vi "Velocity_Trajectory2.vi"() -> ()   [LabVIEW 2017]
uses:
  <vilib>/Analysis/1siggen.llb/Ramp Pattern by Samples.vi
  <vilib>/Analysis/NI_AALBase.lvlib
panel:
  in  "Max Velocity":dbl=2.0
  in  "Theta Final":dbl=100.0
  in  "Theta Initial":dbl=50.0
  out "Waveform Graph":dbl[](graph)=[0.0, 0.010101010101010102, 0.020202020202020204, 0.030303030303030304, 0.04040404040404041, 0.05050505050505051, 0.060606060606060615, 0.07070707070707072, 0.08080808080808081, 0.09090909090909091, 0.10101010101010101, 0.1111111111111111, 0.1212121212121212, 0.1313131313131313, 0.1414141414141414, 0.15151515151515152, 0.16161616161616163, 0.17171717171717174, 0.18181818181818185, 0.19191919191919196, 0.20202020202020207, 0.21212121212121218, 0.2222222222222223, 0.2323232323232324, 0.24242424242424251, 0.2525252525252526, 0.2626262626262627, 0.2727272727272728, 0.28282828282828293, 0.29292929292929304, 0.30303030303030315, 0.31313131313131326, 0.32323232323232337, 0.3333333333333335, 0.3434343434343436, 0.3535353535353537, 0.3636363636363638, 0.3737373737373739, 0.38383838383838403, 0.39393939393939414, 0.40404040404040426, 0.41414141414141437, 0.4242424242424245, 0.4343434343434346, 0.4444444444444447, 0.4545454545454548, 0.4646464646464649, 0.47474747474747503, 0.48484848484848514, 0.49494949494949525, 0.5050505050505053, 0.5151515151515154, 0.5252525252525254, 0.5353535353535355, 0.5454545454545455, 0.5555555555555556, 0.5656565656565656, 0.5757575757575757, 0.5858585858585857, 0.5959595959595958, 0.6060606060606059, 0.6161616161616159, 0.626262626262626, 0.636363636363636, 0.6464646464646461, 0.6565656565656561, 0.6666666666666662, 0.6767676767676762, 0.6868686868686863, 0.6969696969696964, 0.7070707070707064, 0.7171717171717165, 0.7272727272727265, 0.7373737373737366, 0.7474747474747466, 0.7575757575757567, 0.7676767676767667, 0.7777777777777768, 0.7878787878787868, 0.7979797979797969, 0.808080808080807, 0.818181818181817, 0.8282828282828271, 0.8383838383838371, 0.8484848484848472, 0.8585858585858572, 0.8686868686868673, 0.8787878787878773, 0.8888888888888874, 0.8989898989898975, 0.9090909090909075, 0.9191919191919176, 0.9292929292929276, 0.9393939393939377, 0.9494949494949477, 0.9595959595959578, 0.9696969696969678, 0.9797979797979779, 0.989898989898988, 0.999999999999998, 1.0, 1.0, 1.0, 1.0, 1.0, 1.0, 1.0, 1.0, 1.0, 1.0, 1.0, 1.0, 1.0, 1.0, 1.0, 1.0, 1.0, 1.0, 1.0, 1.0, 1.0, 1.0, 1.0, 1.0, 1.0, 1.0, 1.0, 1.0, 1.0, 1.0, 1.0, 1.0, 1.0, 1.0, 1.0, 1.0, 1.0, 1.0, 1.0, 1.0, 1.0, 1.0, 1.0, 1.0, 1.0, 1.0, 1.0, 1.0, 1.0, 1.0, 1.0, 1.0, 1.0, 1.0, 1.0, 1.0, 1.0, 1.0, 1.0, 1.0, 1.0, 1.0, 1.0, 1.0, 1.0, 1.0, 1.0, 1.0, 1.0, 1.0, 1.0, 1.0, 1.0, 1.0, 1.0, 1.0, 1.0, 1.0, 1.0, 1.0, 1.0, 1.0, 1.0, 1.0, 1.0, 1.0, 1.0, 1.0, 1.0, 1.0, 1.0, 1.0, 1.0, 1.0, 1.0, 1.0, 1.0, 1.0, 1.0, 1.0, 1.0, 0.98989898989899, 0.9797979797979799, 0.9696969696969698, 0.9595959595959598, 0.9494949494949497, 0.9393939393939397, 0.9292929292929296, 0.9191919191919196, 0.9090909090909095, 0.8989898989898994, 0.8888888888888894, 0.8787878787878793, 0.8686868686868693, 0.8585858585858592, 0.8484848484848492, 0.8383838383838391, 0.8282828282828291, 0.818181818181819, 0.808080808080809, 0.7979797979797989, 0.7878787878787888, 0.7777777777777788, 0.7676767676767687, 0.7575757575757587, 0.7474747474747486, 0.7373737373737386, 0.7272727272727285, 0.7171717171717185, 0.7070707070707084, 0.6969696969696983, 0.6868686868686883, 0.6767676767676782, 0.6666666666666682, 0.6565656565656581, 0.6464646464646481, 0.636363636363638, 0.626262626262628, 0.6161616161616179, 0.6060606060606079, 0.5959595959595978, 0.5858585858585877, 0.5757575757575777, 0.5656565656565676, 0.5555555555555576, 0.5454545454545475, 0.5353535353535375, 0.5252525252525274, 0.5151515151515174, 0.5050505050505073, 0.4949494949494972, 0.4848484848484871, 0.47474747474747697, 0.46464646464646686, 0.45454545454545675, 0.44444444444444664, 0.43434343434343653, 0.4242424242424264, 0.4141414141414163, 0.4040404040404062, 0.3939393939393961, 0.383838383838386, 0.37373737373737587, 0.36363636363636576, 0.35353535353535565, 0.34343434343434553, 0.3333333333333354, 0.3232323232323253, 0.3131313131313152, 0.3030303030303051, 0.292929292929295, 0.28282828282828487, 0.27272727272727476, 0.26262626262626465, 0.25252525252525454, 0.24242424242424443, 0.23232323232323432, 0.2222222222222242, 0.2121212121212141, 0.202020202020204, 0.19191919191919388, 0.18181818181818377, 0.17171717171717366, 0.16161616161616355, 0.15151515151515343, 0.14141414141414332, 0.1313131313131332, 0.12121212121212312, 0.11111111111111302, 0.10101010101010292, 0.09090909090909283, 0.08080808080808273, 0.07070707070707263, 0.06060606060606253, 0.050505050505052426, 0.04040404040404232, 0.030303030303032222, 0.020202020202022122, 0.01010101010101202, 1.9194630558388645e-15, 0.0, 0.0, 0.0, 0.0, 0.0, 0.0, 0.0, 0.0, 0.0, 0.0, 0.0, 0.0, 0.0, 0.0, 0.0, 0.0, 0.0, 0.0, 0.0, 0.0, 0.0, 0.0, 0.0, 0.0, 0.0, 0.0, 0.0, 0.0, 0.0, 0.0, 0.0, 0.0, 0.0, 0.0, 0.0, 0.0, 0.0, 0.0, 0.0, 0.0, 0.0, 0.0, 0.0, 0.0, 0.0, 0.0, 0.0, 0.0, 0.0, 0.0, 0.0, 0.0, 0.0, 0.0, 0.0, 0.0, 0.0, 0.0, 0.0, 0.0, 0.0, 0.0, 0.0, 0.0, 0.0, 0.0, 0.0, 0.0, 0.0, 0.0, 0.0, 0.0, 0.0, 0.0, 0.0, 0.0, 0.0, 0.0, 0.0, 0.0, 0.0, 0.0, 0.0, 0.0, 0.0, 0.0, 0.0, 0.0, 0.0, 0.0, 0.0, 0.0, 0.0, 0.0, 0.0, 0.0, 0.0, 0.0, 0.0, 0.0]
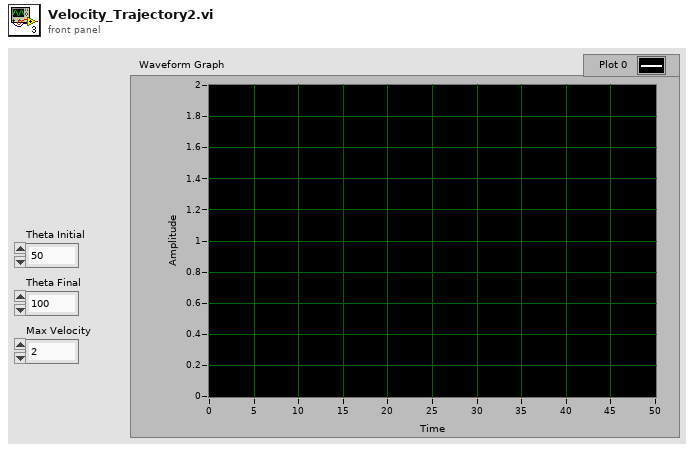
[diagram p1: front panel]
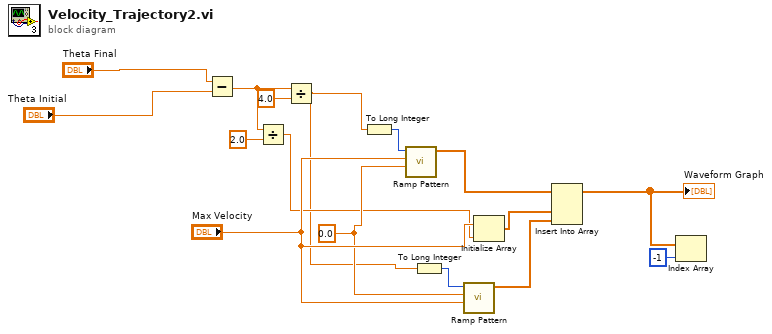
[diagram p0: block diagram]
diagram:
  w13 = 0.0
  n1 = Subtract(x="Theta Final", y="Theta Initial") -> (x-y=w5:dbl)
  n2 = Divide(x=w5, y=2.0) -> (x/y=w4:dbl)
  n3 = Divide(x=w5, y=4.0) -> (x/y=w3:dbl)
  n4 = To Long Integer(number=w3) -> (32bit integer=w7:i32)
  n5 = call-poly <vilib>:"Ramp Pattern.vi"("start"=w13, "end"="Max Velocity", "samples"=w7) -> ("Ramp Pattern"=w16:dbl[])  [unwired: 7 in, 1 out]
  n6 = To Long Integer(number=w3) -> (32bit integer=w6:i32)
  n7 = call-poly <vilib>:"Ramp Pattern.vi"("start"="Max Velocity", "end"=w13, "samples"=w6) -> ("Ramp Pattern"=w10:dbl[])  [unwired: 7 in, 1 out]
  n8 = Initialize Array("Max Velocity", w4) -> (w15:dbl[])
  n9 = Insert Into Array(array=w16, new element #1=w15, new element #2=w10) -> (w12:dbl[])  [unwired: 1 in]
  "Waveform Graph" <- w12
  n10 = Index Array(array=w12, index=-1) -> ()  [unwired: 1 out]
